vi "DefenseCrosser.vi"(6 "FirstTime?":bool, 7 "Wait Time":dbl, 8 "Roll":dbl, 9 "Pitch":dbl, 10 "RightIn":dbl, 11 "LeftIn":dbl) -> (0 "Complete?":bool, 2 "RightOut":dbl, 3 "LeftOut":dbl)   [LabVIEW 2015]
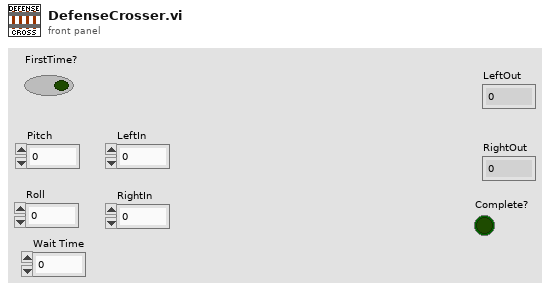
[diagram p1: front panel]
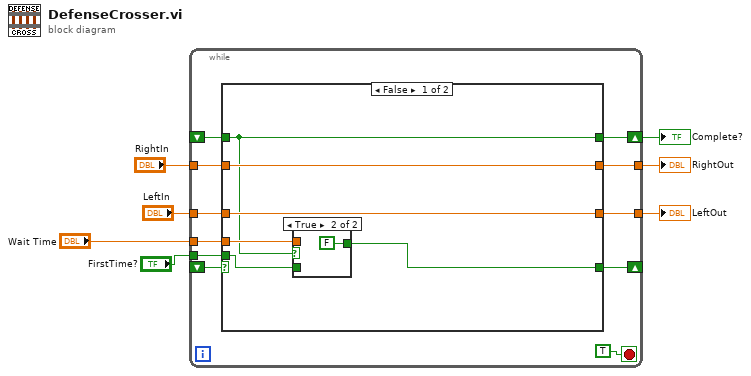
[diagram p0: block diagram]
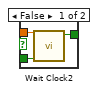
[diagram p2: hidden frame]
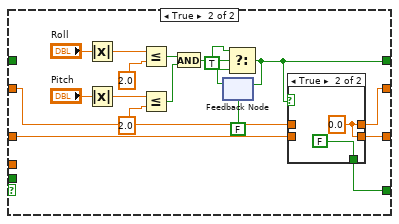
[diagram p3: hidden frame]
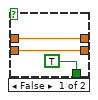
[diagram p4: hidden frame]
diagram:
  n1 = while {
    tunnel: "FirstTime?" -> [w18]
    shift-right: [w16] -> _
    shift-left: _ -> [w17]
    tunnel: "LeftIn" -> [w14]
    tunnel: [w13] -> w5
    tunnel: "RightIn" -> [w12]
    tunnel: [w11] -> w3
    tunnel: "Wait Time" -> [w10]
    shift-right: [w9] -> w1
    shift-left: _ -> [w8]
    stop <- TRUE stop-if-true
    n2 = case shown="False" w17 {
      tunnel: w18 -> [w24 _]
      tunnel: [w23 w30] -> w16
      tunnel: [w22 w45] -> w13
      tunnel: w14 -> [w22 w46]
      tunnel: w12 -> [w21 w43]
      tunnel: [w21 w44] -> w11
      tunnel: w10 -> [w20 _]
      tunnel: [w19 w29] -> w9
      tunnel: w8 -> [w19 _]
      frame False {
        n3 = case shown="True" w19 {
          tunnel: w24 -> [w27 _]
          tunnel: [w26 FALSE ("Completed")] -> w23
          tunnel: w20 -> [w25 _]
          frame False {
            n4 = call "Wait Clock2.vi"("First Time?"=w27, "Target Time"=w25) -> ("Completed"=w26:bool)  [unwired: 9 in]
          }
          frame True {
          }
        }
      }
      frame True {
        n5 = Absolute Value(x="Roll") -> (abs(x)=w36:dbl)
        n6 = Absolute Value(x="Pitch") -> (abs(x)=w35:dbl)
        n7 = Less Or Equal?(x=w36, y=2.0) -> (x <= y?=w32:bool)
        n8 = Less Or Equal?(x=w35, y=2.0) -> (x <= y?=w31:bool)
        n9 = And(x=w32, y=w31) -> (x .and. y?=w42:bool)
        n10 = feedback #1(FALSE) -> (w40:bool)
        n11 = Select(t=TRUE, s=w42, f=w40) -> (s? t:f=w29:bool)
        n12 = feedback-in #1(w29) -> ()
        n13 = case shown="True" w29 {
          tunnel: [w49 w51] -> w45
          tunnel: w46 -> [w49 _]
          tunnel: [w48 w51] -> w44
          tunnel: w43 -> [w48 _]
          tunnel: [TRUE ("Completed") FALSE ("Completed")] -> w30
          frame False {
          }
          frame True {
            w51 = 0.0 ("LeftIn")
          }
        }
      }
    }
  }
  "LeftOut" <- w5
  "RightOut" <- w3
  "Complete?" <- w1
